vi "Waveform-GetAttributes.vi"(8 "error in (no error)":errorcluster, 11 "signal in":waveform(dbl)) -> (0 "error out":errorcluster, 2 "WaveformInfo":T1, 3 "signal out":waveform(dbl))   [LabVIEW 2020, in "CSM-TagRouter.lvlib"]
uses:
  CSM-TagRouter.lvlib
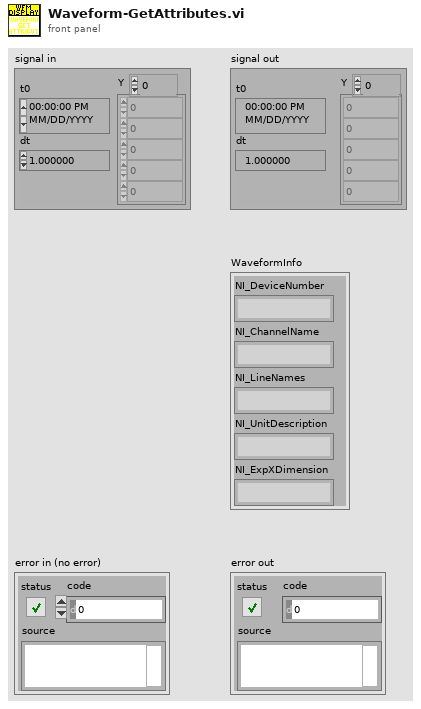
[diagram p1: front panel]
types:
  T1 = cluster{"NI_DeviceNumber":string, "NI_ChannelName":string, "NI_LineNames":string, "NI_UnitDescription":string, "NI_ExpXDimension":string}
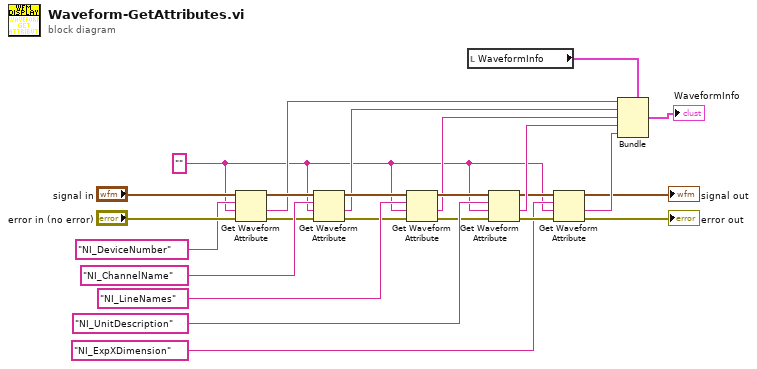
[diagram p0: block diagram]
diagram:
  w4 = "" ("name")
  n1 = Get Waveform Attribute(4:"error in (no error)", 5:w4, 6:"NI_DeviceNumber" ("name"), 7:"signal in") -> (0:w18:errorcluster, 1:w13:string, 3:w19:waveform(dbl))  [unwired: 1 out]
  n2 = Get Waveform Attribute(4:w18, 5:w4, 6:"NI_ChannelName" ("name"), 7:w19) -> (0:w16:errorcluster, 1:w12:string, 3:w17:waveform(dbl))  [unwired: 1 out]
  n3 = Get Waveform Attribute(4:w16, 5:w4, 6:"NI_LineNames" ("name"), 7:w17) -> (0:w14:errorcluster, 1:w11:string, 3:w15:waveform(dbl))  [unwired: 1 out]
  n4 = local read "WaveformInfo"() -> (w9:T1)
  n5 = Get Waveform Attribute(4:w14, 5:w4, 6:"NI_UnitDescription" ("name"), 7:w15) -> (0:w8:errorcluster, 1:w7:string, 3:w6:waveform(dbl))  [unwired: 1 out]
  n6 = Get Waveform Attribute(4:w8, 5:w4, 6:"NI_ExpXDimension" ("name"), 7:w6) -> (0:→"error out":errorcluster, 1:w3:string, 3:→"signal out":waveform(dbl))  [unwired: 1 out]
  n7 = Bundle(cluster=w9, "NI_DeviceNumber"=w13, "NI_ChannelName"=w12, "NI_LineNames"=w11, "NI_UnitDescription"=w7, "NI_ExpXDimension"=w3) -> (→"WaveformInfo":T1)
